vi "testSensorNameToId.vi"(8 "error in (no error)":errorcluster) -> (0 "error out":errorcluster)   [LabVIEW 2016]
doc: "Test the to map the abbreviated sensor name to sensor Id."
uses:
  <vilib>/addons/_JKI Toolkits/Caraya/classes/Test/Test.lvclass
  <vilib>/addons/_JKI Toolkits/Caraya/classes/Assert/Assert.lvclass
  MatOper/MatOper.lvclass
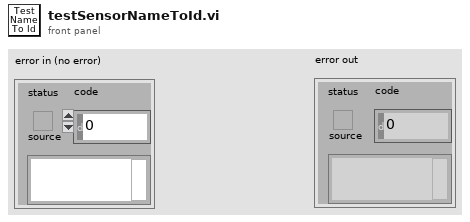
[diagram p1: front panel]
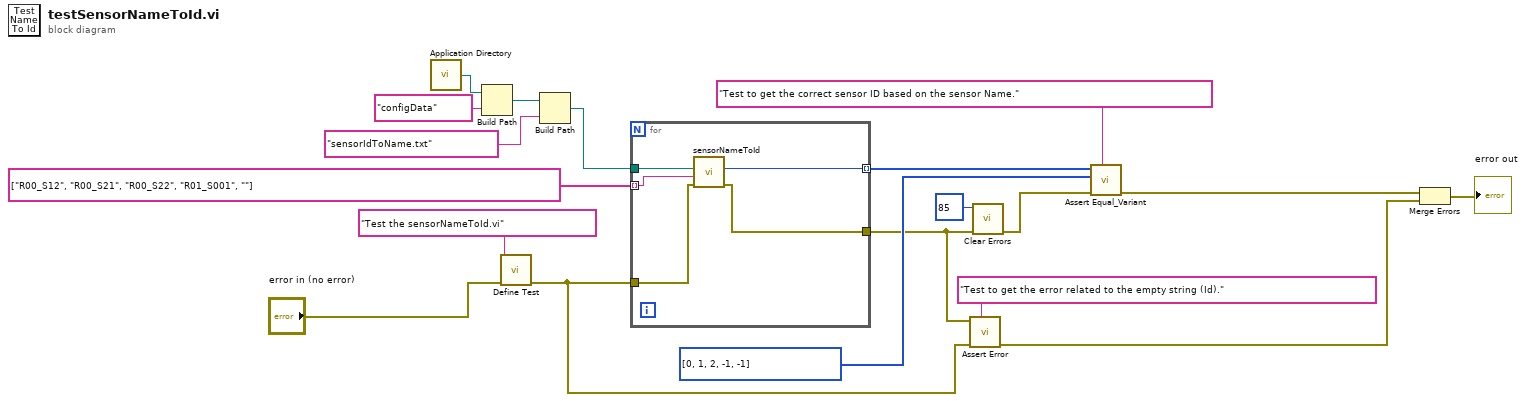
[diagram p0: block diagram]
diagram:
  n1 = call <vilib>:"Application Directory.vi"() -> ("Application Directory"=w18:path)
  n2 = Build Path(base path=w18, name or relative path="configData") -> (appended path=w16:path)
  n3 = call <vilib>:"Define Test.vi"("error in (no error)"="error in (no error)", "Label (VI Title)"="Test the sensorNameToId.vi") -> ("error out"=w8:errorcluster)  [unwired: 9 in]
  n4 = Build Path(base path=w16, name or relative path="sensorIdToName.txt") -> (appended path=w14:path)
  n5 = for {
    tunnel: w14 -> [w24]
    tunnel: w8 -> [w23]
    tunnel: [w20] -> w6
    tunnel: string[] ["R00_S12", "R00_S21", "R00_S22", "R01_S001", ""] -> [w22] mode=indexing
    tunnel: [w21] -> w10 mode=indexing
    n6 = call "sensorNameToId.vi"("error in (no error)"=w23, "Sensor Name"=w22, "Path"=w24) -> ("error out"=w20:errorcluster, "Sensor ID"=w21:i32)  [unwired: 6 in, 1 out]
  }
  n7 = call <vilib>:"Assert Error.vi"("Label"="Test to get the error related to the empty string (Id).", "error in (no error)"=w8, "Error?"=w6) -> ("error out"=w3:errorcluster)  [unwired: 8 in]
  n8 = call <vilib>:"Clear Errors.vi"("error in (no error)"=w6, "specific error code to clear (0: all)"=85) -> ("error out"=w7:errorcluster)  [unwired: 4 in, 1 out]
  n9 = call <vilib>:"Assert Equal_Variant.vi"("Label"="Test to get the correct sensor ID based on the sensor Name." ("Label (VI Title)"), "error in (no error)"=w7, "Y"=i32[] [0, 1, 2, -1, -1], "X"=w10) -> ("error out"=w4:errorcluster)  [unwired: 7 in]
  n10 = Merge Errors(w4, w3) -> (→"error out":errorcluster)
